vi "Write Enable.vi"(8 "error in (no error)":errorcluster, 10 "Enable":bool, 11 "JsonReportPlugin in":refnum<class "JsonReportPlugin.lvclass">) -> (0 "error out":errorcluster, 3 "JsonReportPlugin out":refnum<class "JsonReportPlugin.lvclass">)   [LabVIEW 2015, in "JsonReportPlugin.lvclass"]
uses:
  JsonReportPlugin.lvclass
  JsonReportPlugin.lvclass/JsonReportPlugin.ctl
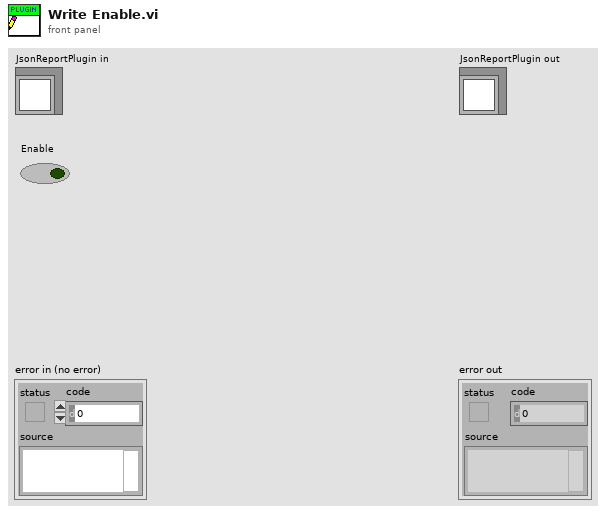
[diagram p1: front panel]
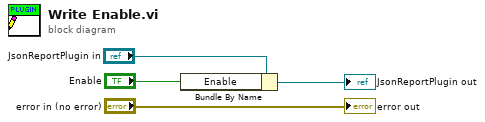
[diagram p0: block diagram]
diagram:
  n1 = Bundle By Name(cluster="JsonReportPlugin in", "Enable"="Enable") -> (→"JsonReportPlugin out":refnum<class "JsonReportPlugin.lvclass">)
  "error out" <- "error in (no error)"
